vi "AOL driver.vi"(8 "Error in":errorcluster, 9 "Acquired z-plane index / volume index":i32, 11 "AOL_Globals":T1={"Imaging Protocol"=enum."AOL Z-Stack", "Number of POI"=0, "Number of Miniscans"=0, "Number of Trials"=0, "Number of Cycles "=0, "# Averaged Frames"=0, "Laser power (%)"=0, "Pockels"=0.0, "Acquisition Length (sec)"=0.0, "Fill time (us)"=0.0, "POI Dwell time (us)"=0.0, "Miniscan Dwell time per pixel (us)"=0.0, "PMT 1"=0.0, "PMT 2"=0.0, "Back Apperture"=200.0, "Frame Size"=0, "Center Frequency"=0.0, "Field of View"=0.0, "DwellTime (us)"=0.0, "Wavelength (nm)"=0.0, "Zoom"=0.0, "AOL Z"=0.0, "AOL Mode"=enum."Raster", "GridXY"=0.0, "GridZ"=0.0, "TriggerPeriod (sec)"=0.0, "Number of Pixels in Miniscan"=0, "Experiment folder path"=path "", "X centre"=0.0, "Y centre"=0.0, "Angle (degrees)"=0.0, "Plane Mode"=0, "Threshold"=[], "Regenerate Chirps"=FALSE, "Rectangle ROI length (pixels)"=0, "Rectangle ROI height (pixels)"=0, "AOD fill"=0, "Samples Wait after Trigger"=0, "StartUp Delay"=0, "Slip Cycle"=163840, "Add Cycle"=FALSE} {"Plane Mode" items=["XY Plane"]; "Frame Size" items=["100X100"=100, "128X128"=128, "200X200"=200, "256X256"=256, "512X512"=512, "1024x1024"=1024, "2048x2048"=2048]; "Back Apperture" format="%#.6g"; "Pockels" format="%#.6g"; "PMT 2" format="%#.6g"; "PMT 1" format="%#.6g"; "Angle (degrees)" format="%#.6g"; "POI Dwell time (us)" format="%#.6g"}) -> (0 "Error out":errorcluster)   [LabVIEW 2013]
uses:
  Typedefs/Controls/AOL_Globals.ctl
  Typedefs/Imaging Protocols enum.ctl
  Typedefs/Frame Size.ctl
  Typedefs/AOL modes.ctl
  Typedefs/Plane Mode.ctl
  Typedefs/Read Write Enum.ctl
panel:
  out "execution time (ms)":u32
  out "Time per plane":u32
  # "<--- around 15ms max"
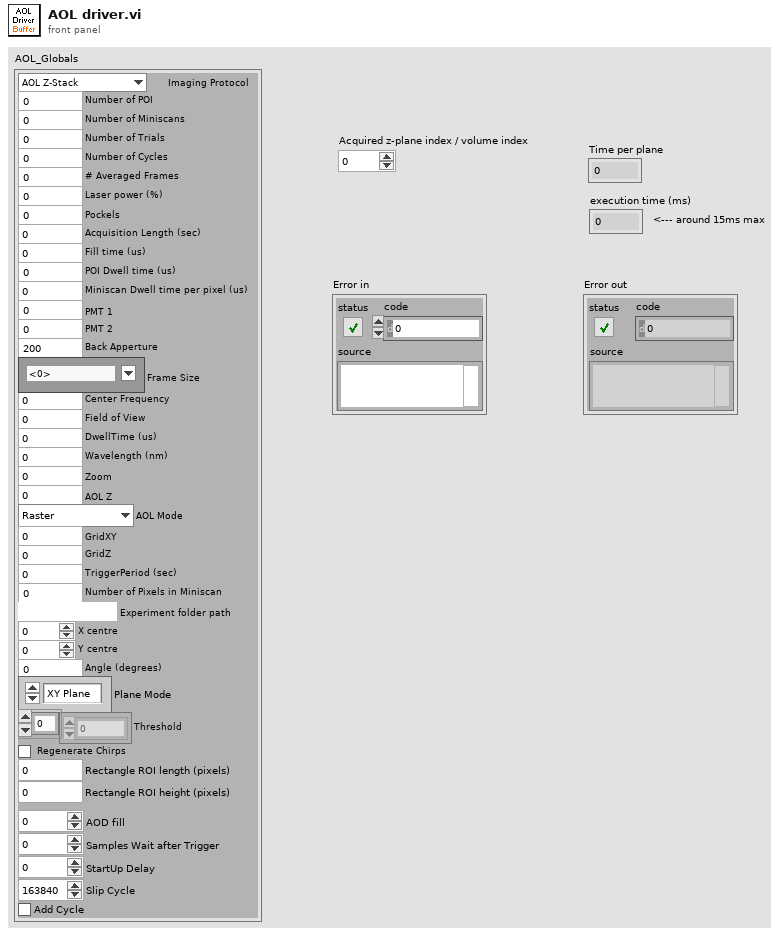
[diagram p1: front panel]
types:
  T1 = typedef "AOL_Globals.ctl" = cluster{"Imaging Protocol":T2, "Number of POI":u16, "Number of Miniscans":u16, "Number of Trials":u16, "Number of Cycles ":u64, "# Averaged Frames":u16, "Laser power (%)":u8, "Pockels":dbl, "Acquisition Length (sec)":dbl, "Fill time (us)":dbl, "POI Dwell time (us)":dbl, "Miniscan Dwell time per pixel (us)":dbl, "PMT 1":dbl, "PMT 2":dbl, "Back Apperture":dbl, "Frame Size":T3, "Center Frequency":dbl, "Field of View":dbl, "DwellTime (us)":dbl, "Wavelength (nm)":dbl, "Zoom":dbl, "AOL Z":dbl, "AOL Mode":T4, "GridXY":dbl, "GridZ":dbl, "TriggerPeriod (sec)":dbl, "Number of Pixels in Miniscan":u16, "Experiment folder path":path, "X centre":dbl, "Y centre":dbl, "Angle (degrees)":dbl, "Plane Mode":T5, "Threshold":u16[], "Regenerate Chirps":bool, "Rectangle ROI length (pixels)":u16, "Rectangle ROI height (pixels)":u16, "AOD fill":u16, "Samples Wait after Trigger":u16, "StartUp Delay":i32, "Slip Cycle":u32, "Add Cycle":bool}
  T2 = typedef "Imaging Protocols enum.ctl" = enum16{"AOL Z-Stack", "Motor Z Stack", "Functional Acquisition", "Single Plane Acquisition", "Volume Acquisition", "Live Imaging", "Live Plane Imaging", "Live Volume Imaging"}
  T3 = typedef "Frame Size.ctl" = u16
  T4 = typedef "AOL modes.ctl" = enum16{"Raster", "Structural", "Pointing", "Mini Scan", "Alignment"}
  T5 = typedef "Plane Mode.ctl" = u16
  T6 = typedef "Read Write Enum.ctl" = enum16{"Read", "Write"}
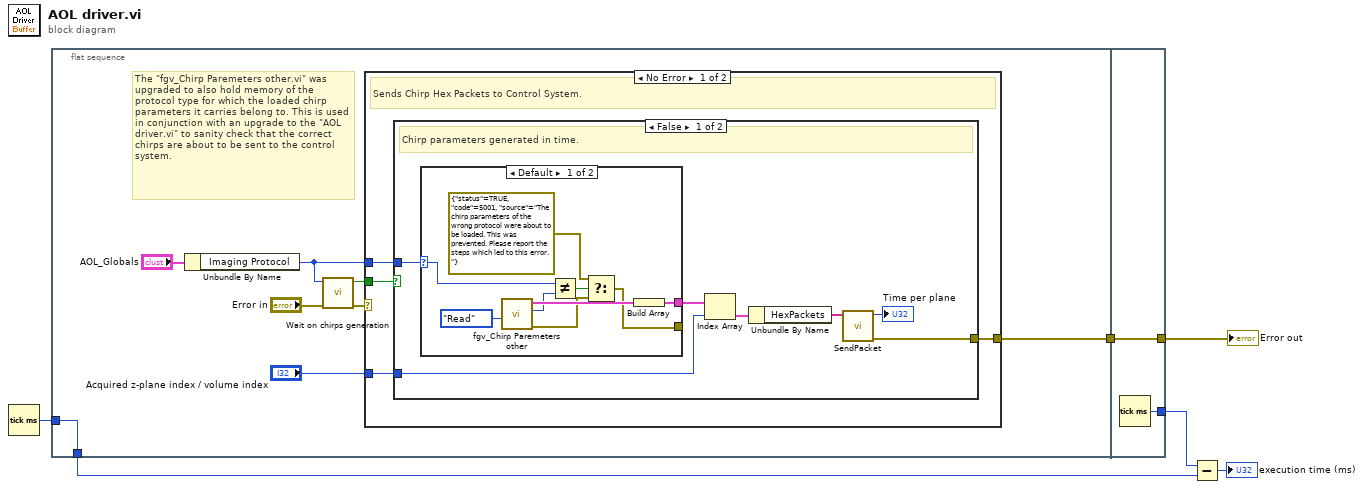
[diagram p0: block diagram]
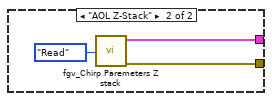
[diagram p2: hidden frame]
diagram:
  n1 = Tick Count (ms)() -> (millisecond timer value=w6:u32)
  n2 = flat-sequence {
    tunnel: w6 -> [w11]
    tunnel: [w11] -> w4
    tunnel: [w7] -> w1
    tunnel: [w40] -> w3
    tunnel: [w39] -> w2
    tunnel: w1 -> [w39]
    frame #0 {
      # "The \"fgv_Chirp Paremeters other.vi\" was upgraded to also hold memory of the protocol type for which the loaded chirp parameters it carries belong to. This is used in conjunction with an upgrade to the \"AOL driver.vi\" to sanity check that the correct chirps are about to be sent to the control system."
      n3 = Unbundle By Name("AOL_Globals") -> ("Imaging Protocol"=w8:T2)
      n4 = call "Wait on chirps generation.vi"("error in (no error)"="Error in", "Imaging Protocol"=w8) -> ("error out"=w14:errorcluster, "Timed out waiting on Chirps generation"=w10:bool)  [unwired: 8 in]
      n5 = case shown="No Error" w14 {
        selector: w14 -> [_ w38]
        tunnel: [w18 w38] -> w7
        tunnel: "Acquired z-plane index / volume index" -> [w17 _]
        tunnel: w10 -> [w16 _]
        tunnel: w8 -> [w15 _]
        frame No Error {
          # "Sends Chirp Hex Packets to Control System."
          n6 = case shown="False" w16 {
            tunnel: [w25 _] -> w18
            tunnel: w17 -> [w24 _]
            tunnel: w15 -> [w19 _]
            frame False {
              # "Chirp parameters generated in time."
              n7 = case shown="Default" w19 {
                selector: w19 -> [w30 _]
                tunnel: [w32 w36] -> w20
                tunnel: [w27 w35] -> _
                frame Default {
                  n8 = call "fgv_Chirp Paremeters other.vi"("Function"=Read_Write_Enum."Read") -> ("error out"=w28:errorcluster, "Imaging Protocol"=w31:T2, "Chirps"=w33:cluster{"HexPackets":string[]})  [unwired: 8 in]
                  n9 = Not Equal?(x=w30, y=w31) -> (x != y?=w29:bool)
                  n10 = Select(t=errorcluster {"status"=TRUE, "code"=5001, "source"="The chirp parameters of the wrong protocol were about to be loaded. This was prevented. Please report the steps which led to this error."}, s=w29, f=w28) -> (s? t:f=w27:errorcluster)
                  n11 = Build Array(w33) -> (w32:cluster{"HexPackets":string[]}[])
                }
                frame "AOL Z-Stack" {
                  n12 = call "fgv_Chirp Paremeters Z stack.vi"("Function"=Read_Write_Enum."Read") -> ("error out"=w35:errorcluster, "Z-stack Chirp parameters (all Z planes)"=w36:cluster{"HexPackets":string[]}[])  [unwired: 9 in]
                }
              }
              n13 = Index Array(array=w20, index=w24) -> (element=w23:cluster{"HexPackets":string[]})
              n14 = Unbundle By Name(w23) -> ("HexPackets"=w22:string[])
              n15 = call "SendPacket.vi"("Packet Array"=w22) -> ("error out"=w25:errorcluster, "Time per plane"=→"Time per plane":u32)  [unwired: 9 in]
            }
            frame True {
              # "Timed out waiting on chirp parameters generation."
            }
          }
        }
        frame Error {
        }
      }
    }
    frame #1 {
      n16 = Tick Count (ms)() -> (millisecond timer value=w40:u32)
    }
  }
  n17 = Subtract(x=w3, y=w4) -> (x-y=→"execution time (ms)":u32)
  "Error out" <- w2
